vi "read_rn16_v0.vi"() -> ()   [LabVIEW 2015]
panel:
  out "Array 2":dbl[](array[numeric])
  out "Array":dbl[](array[numeric])
  out "Signals":dynamicdata(graph)
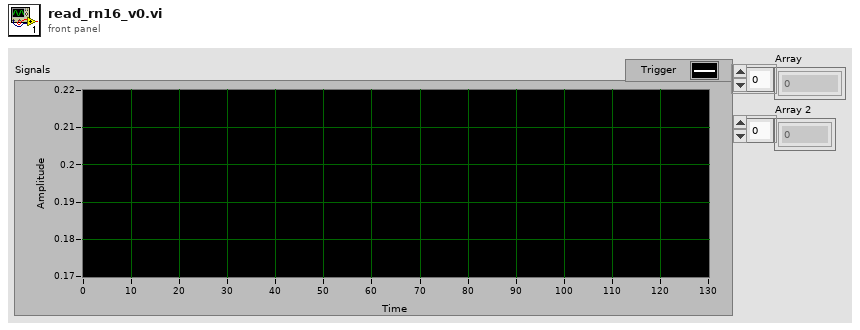
[diagram p1: front panel]
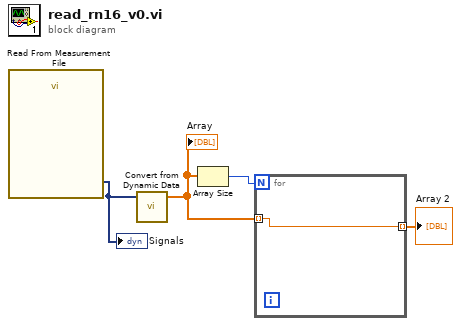
[diagram p0: block diagram]
diagram:
  n1 = call "Read From Measurement File"() -> ("Signals"=w4:dynamicdata)  [unwired: 6 in, 5 out]
  "Signals" <- w4
  n2 = call "Convert from Dynamic Data"("Dynamic Data Type"=w4) -> ("Array"=w2:dbl[])  [unwired: 3 in]
  "Array" <- w2
  n3 = Array Size(array=w2) -> (size(s)=w3:i32)
  n4 = for {
    N: w3 -> [_]
    tunnel: w2 -> [w5] mode=indexing
    tunnel: [w5] -> w1 mode=indexing
  }
  "Array 2" <- w1
